vi "Fill Map with Distance.vi"(8 "error in (no error)":errorcluster, 11 "Grassfire Algorithm in":refnum<class "Grassfire Algorithm.lvclass">) -> (0 "error out":errorcluster, 3 "Grassfire Algorithm out":refnum<class "Grassfire Algorithm.lvclass">)   [LabVIEW 2019, in "Grassfire Algorithm.lvclass"]
uses:
  Grassfire Algorithm.lvclass
  Index Column Row--cluster.ctl
  Grassfire Algorithm.lvclass/Grassfire Algorithm.ctl
panel:
  out "i":i32
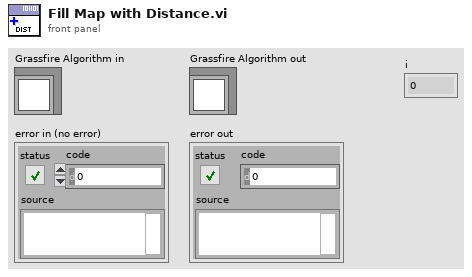
[diagram p1: front panel]
types:
  T1 = typedef "Grassfire Algorithm.lvclass/Index Column Row--cluster.ctl" = cluster{"Row":i32, "Column":i32}
  T2 = typedef "Grassfire Algorithm.lvclass/Solution Grid Cell Private--cluster.ctl" = cluster{"Picture":T3, "Value":dbl}
  T3 = typedef "Grassfire Algorithm.lvclass/Solution--picture ring.ctl" = i64
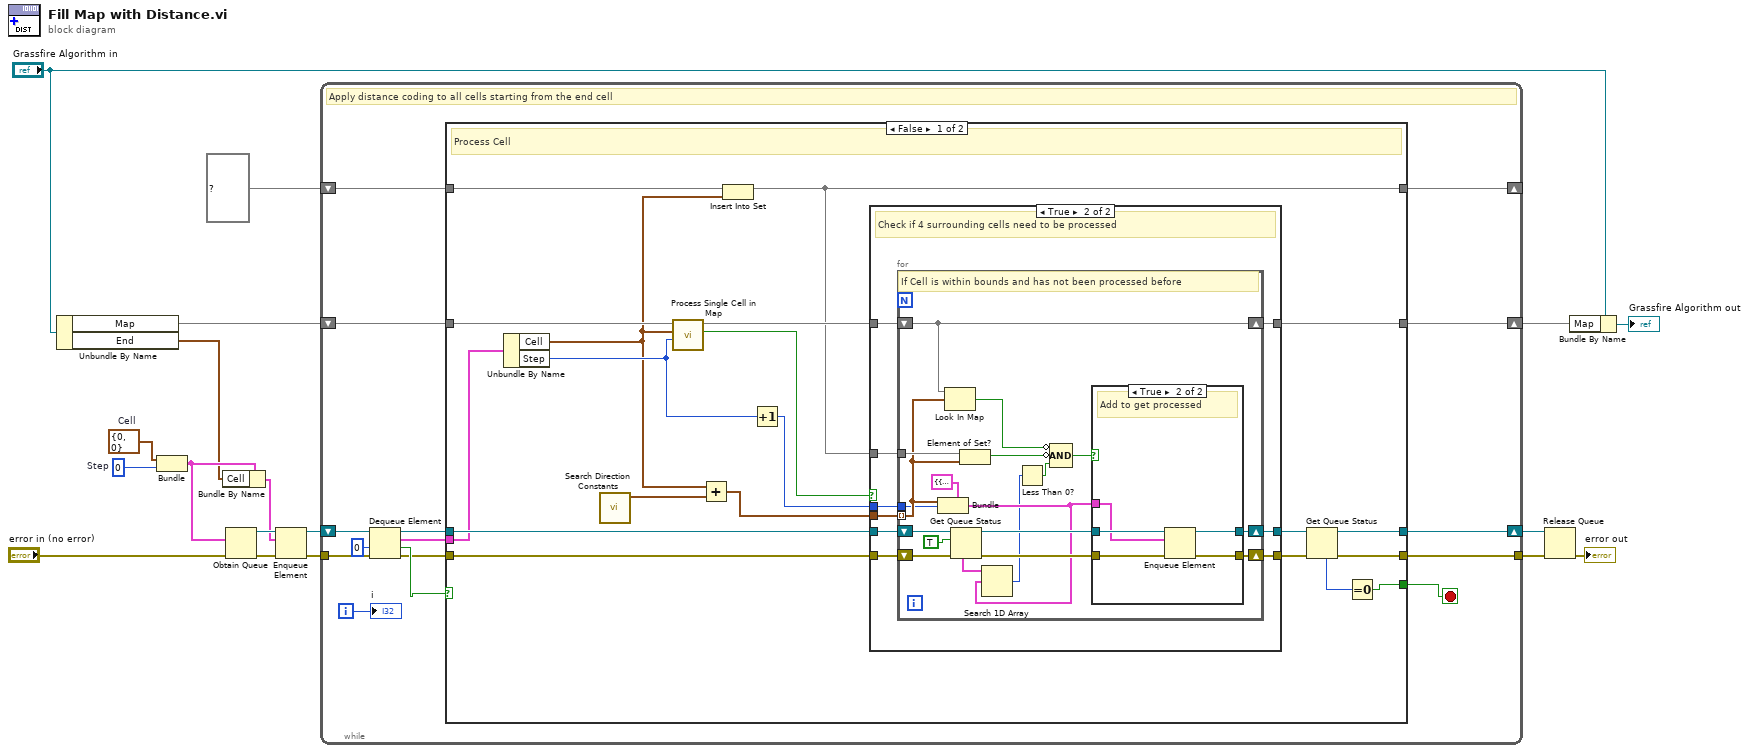
[diagram p0: block diagram]
diagram:
  w5 = T1 {"Row"=0, "Column"=0}  # Cell
  w4 = 0  # Step
  n1 = Unbundle By Name("Grassfire Algorithm in") -> ("Map"=w15:map{T1, T2}, "End"=w2:T1)
  n2 = Bundle("Cell"=w5, "Step"=w4) -> (w3:cluster{"Cell":T1, "Step":i32})  [unwired: 1 in]
  n3 = Bundle By Name(cluster=w3, "Cell"=w2) -> (w1:cluster{"Cell":T1, "Step":i32})
  n4 = Obtain Queue(element data type=w3, error in (no error)="error in (no error)") -> (queue out=w13:refnum<queue>, error out=w11:errorcluster)  [unwired: 3 in, 1 out]
  n5 = Enqueue Element(queue=w13, element=w1, error in (no error)=w11) -> (queue out=w12:refnum<queue>, error out=w8:errorcluster)  [unwired: 1 in, 1 out]
  n6 = while {
    shift-right: [w32] -> w18
    shift-left: w15 -> [w33]
    shift-right: [w22] -> w14
    shift-left: w12 -> [w28]
    tunnel: w8 -> [w25]
    tunnel: [w23] -> w7
    shift-right: [w20] -> _
    shift-left: set{T1} {} ("set") -> [w21]
    i -> [w31]
    stop <- w19 stop-if-true
    # "Apply distance coding to all cells starting from the end cell"
    n7 = Dequeue Element(queue=w28, timeout in ms (-1)=0, error in (no error)=w25) -> (queue out=w26:refnum<queue>, element=w27:cluster{"Cell":T1, "Step":i32}, timed out?=w29:bool, error out=w24:errorcluster)
    n8 = case shown="False" w29 {
      selector: w29 -> [_ w92]
      tunnel: w33 -> [w53 w96]
      tunnel: [w49 w96] -> w32
      tunnel: w27 -> [w43 _]
      tunnel: w26 -> [w51 w95]
      tunnel: [w35 w95] -> w22
      tunnel: w24 -> [w50 w94]
      tunnel: [w36 w94] -> w23
      tunnel: w21 -> [w47 w93]
      tunnel: [w46 w93] -> w20
      tunnel: [w34 w92] -> w19
      frame False {
        # "Process Cell"
        n9 = Unbundle By Name(w43) -> ("Cell"=w40:T1, "Step"=w42:i32)
        n10 = call "Search Direction Constants.vi"() -> ("Search Direction Cells"=w45:T1[])  [unwired: 10 in, 1 out]
        n11 = call "Process Single Cell in Map.vi"("Step"=w42, "Cell"=w40, "Map in"=w53) -> ("Check Surroundings?"=w52:bool, "Map out"=w48:map{T1, T2})  [unwired: 7 in]
        n12 = Add(x=w40, y=w45) -> (x+y=w44:T1[])
        n13 = Insert Into Set(10:w40, 11:w47) -> (3:w46:set{T1})  [unwired: 1 out]
        n14 = Increment(x=w42) -> (x+1=w41:i32)
        n15 = case shown="True" w52 {
          tunnel: [w55 w64] -> w38
          tunnel: w44 -> [_ w63]
          tunnel: w51 -> [w55 w65]
          tunnel: w50 -> [w54 w62]
          tunnel: [w54 w61] -> w37
          tunnel: [w56 w60] -> w49
          tunnel: w48 -> [w56 w59]
          tunnel: w46 -> [_ w58]
          tunnel: w41 -> [_ w57]
          frame False {
            # "No further actions"
          }
          frame True {
            # "Check if 4 surrounding cells need to be processed"
            n16 = for {
              tunnel: w63 -> [w79] mode=indexing
              shift-right: [w84] -> w64
              shift-left: w65 -> [w76]
              shift-right: [w83] -> w61
              shift-left: w62 -> [w74]
              shift-right: [w77] -> w60
              shift-left: w59 -> [w77]
              tunnel: w58 -> [w80]
              tunnel: w57 -> [w69]
              # "If Cell is within bounds and has not been processed before"
              n17 = Bundle(cluster=cluster{"Cell":T1, "Step":i32} {"Cell"={"Row"=0, "Column"=0}, "Step"=0}, "Cell"=w79, "Step"=w69) -> (w68:cluster{"Cell":T1, "Step":i32})
              n18 = Look In Map(map=w77, key=w79) -> (key not found?=w82:bool)  [unwired: 1 in, 1 out]
              n19 = Get Queue Status(queue=w76, return elements? (F)=TRUE, error in (no error)=w74) -> (queue out=w73:refnum<queue>, error out=w72:errorcluster, elements=w71:cluster{"Cell":T1, "Step":i32}[])  [unwired: 5 out]
              n20 = Element of Set?(10:w79, 11:w80) -> (3:w78:bool)
              n21 = Search 1D Array(1D array=w71, element=w68) -> (index of element=w66:i32)  [unwired: 1 in]
              n22 = Less Than 0?(x=w66) -> (x < 0?=w67:bool)
              n23 = Compound Arithmetic op=AND(invert w82, invert w78, w67) -> (w81:bool)
              n24 = case shown="True" w81 {
                tunnel: w73 -> [w86 w91]
                tunnel: [w86 w90] -> w84
                tunnel: w72 -> [w85 w89]
                tunnel: [w85 w88] -> w83
                tunnel: w68 -> [_ w87]
                frame False {
                  # "Ignore Cell"
                }
                frame True {
                  # "Add to get processed"
                  n25 = Enqueue Element(queue=w91, element=w87, error in (no error)=w89) -> (queue out=w90:refnum<queue>, error out=w88:errorcluster)  [unwired: 1 in, 1 out]
                }
              }
            }
          }
        }
        n26 = Get Queue Status(queue=w38, error in (no error)=w37) -> (queue out=w35:refnum<queue>, error out=w36:errorcluster, # elements in queue=w39:i32)  [unwired: 1 in, 5 out]
        n27 = Equal To 0?(x=w39) -> (x = 0?=w34:bool)
      }
      frame True {
        # "No operations remain"
      }
    }
    "i" <- w31
  }
  n28 = Release Queue(queue=w14, error in (no error)=w7) -> (error out=→"error out":errorcluster)  [unwired: 1 in, 2 out]
  n29 = Bundle By Name(cluster="Grassfire Algorithm in", "Map"=w18) -> (→"Grassfire Algorithm out":refnum<class "Grassfire Algorithm.lvclass">)
